vi "属性节点2.vi"() -> ()   [LabVIEW 2018]
panel:
  in  "枚举":enum16{"A", "V"}(ring)
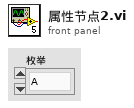
[diagram p1: front panel]
types:
  T1 = enum8{"Enabled", "Disabled", "Disabled and Grayed Out"}
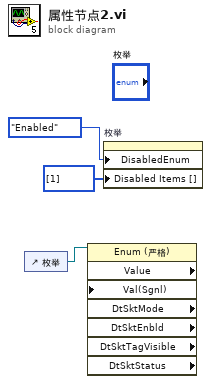
[diagram p0: block diagram]
diagram:
  n1 = control-ref of="枚举"() -> (w2:refnum<vi>)
  n2 = property class="Enum (严格)" props=["Value", "Val(Sgnl)", "DtSktMode", "DtSktEnbld", "DtSktTagVisible", "DtSktStatus"](reference=w2) -> ()  [unwired: 2 in, 7 out]
  n3 = property on="枚举" class="Enum (严格)"("DisabledEnum"=T1."Enabled" ("禁用"), "Disabled Items []"=i32[] [1] ("禁用项[]")) -> ()  [unwired: 2 in, 2 out]
